vi "Produced Methods.vi"(7 "error in":errorcluster) -> (3 "Produced Methods":string[](array[string]), 5 "error out":errorcluster)   [LabVIEW 2012]
uses:
  Folders.ctl
  Design Server.lvlib
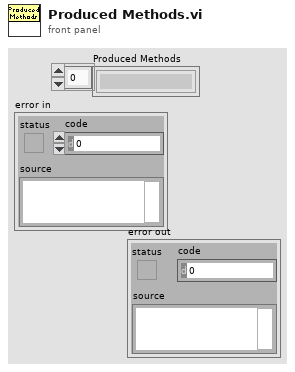
[diagram p1: front panel]
types:
  T1 = typedef "Design Server.lvlib/Folders.ctl" = enum16{"MathcadMethods", "RequestedDesigns", "CompletedDesigns", "MathcadCode", "CollabnetSVN.exe"}
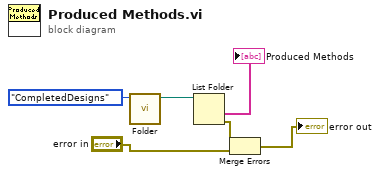
[diagram p0: block diagram]
diagram:
  n1 = call "Folder.vi"("Folders"=Folders."CompletedDesigns") -> ("FolderPath"=w5:path)  [unwired: 8 in, 2 out]
  n2 = List Folder(path=w5) -> (folder names=→"Produced Methods":string[], error out=w3:errorcluster)  [unwired: 3 in, 2 out]
  n3 = Merge Errors(w3, "error in") -> (→"error out":errorcluster)
